vi "Uses Vision.vi"(8 "error in (no error)":errorcluster, 11 "Tosca in":refnum<class "Parameters.lvclass">) -> (0 "error out":errorcluster, 2 "Uses vision":bool, 3 "Tosca out":refnum<class "Parameters.lvclass">)   [LabVIEW 2015, in "Parameters.lvclass"]
uses:
  Parameters.lvclass
  Parameters.lvclass/Parameters.ctl
  Visual Stim VIs/Tosca-Grating Type.ctl
  State/State.lvclass/State.ctl
  State/Read Grating.vi
  State/State.lvclass
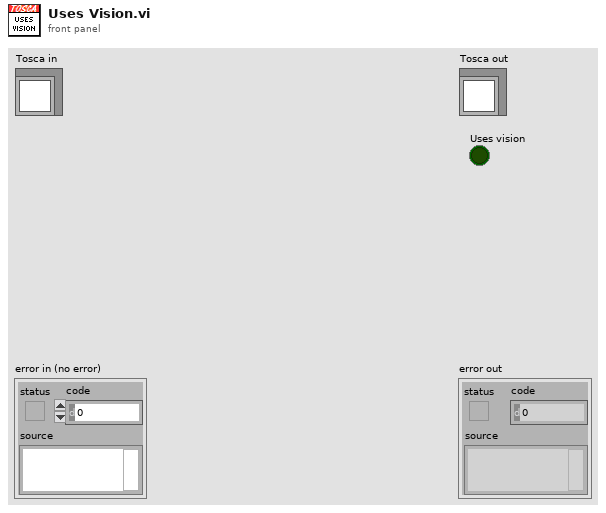
[diagram p1: front panel]
types:
  T1 = typedef "Tosca-Grating Type.ctl" = enum16{"OFF", "Square", "Sine"}
  T2 = typedef "Tosca-Grating.ctl" = cluster{"Type":T1, "Orientation (deg)":dbl, "Spatial frequency (cpd)":dbl, "Velocity (Hz)":dbl, "Contrast":dbl, "Background intensity":dbl, "Duration (ms)":dbl, "Phase (cycles)":dbl}
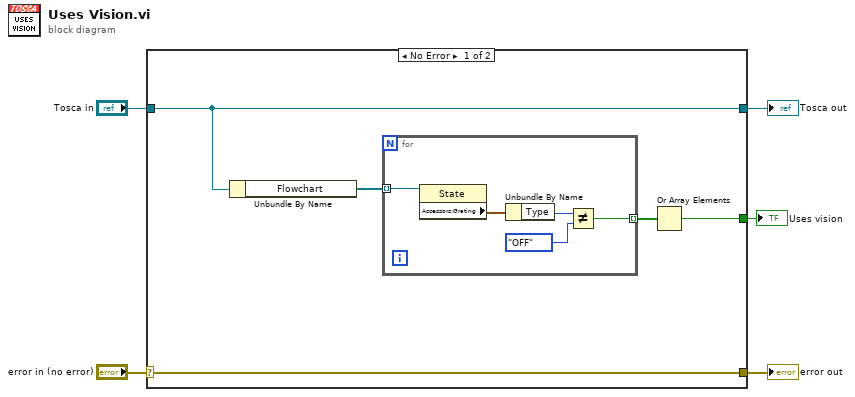
[diagram p0: block diagram]
diagram:
  n1 = case shown="No Error" "error in (no error)" {
    selector: "error in (no error)" -> [w10 w17]
    tunnel: [w10 w17] -> w4
    tunnel: [w9 w16] -> w2
    tunnel: "Tosca in" -> [w9 w16]
    tunnel: [w6 _] -> w1
    frame No Error {
      n2 = Unbundle By Name(w9) -> ("Flowchart"=w8:refnum<class "State.lvclass">[])
      n3 = for {
        tunnel: w8 -> [w15] mode=indexing
        tunnel: [w11] -> w7 mode=indexing
        n4 = property class="State"(reference=w15) -> ("Accessors:Grating"=w14:T2)  [unwired: 1 in, 2 out]
        n5 = Unbundle By Name(w14) -> ("Type"=w13:T1)
        n6 = Not Equal?(x=w13, y=Tosca-Grating_Type."OFF") -> (x != y?=w11:bool)
      }
      n7 = Or Array Elements(Boolean array=w7) -> (logical OR=w6:bool)
    }
    frame Error {
    }
  }
  "error out" <- w4
  "Tosca out" <- w2
  "Uses vision" <- w1
